vi "Write Temperature Control.lvclass.vi"(10 "Temperature Control.lvclass":refnum<class "Temperature Control.lvclass">, 11 "Measurements in":refnum<class "Measurement.lvclass">) -> (3 "Measurements out":refnum<class "Measurement.lvclass">)   [LabVIEW 2020, in "Measurement.lvclass"]
uses:
  Measurement.lvclass
  Instruments/Temperature Control/Temperature Control.lvclass
  Measurement.lvclass/Measurement.ctl
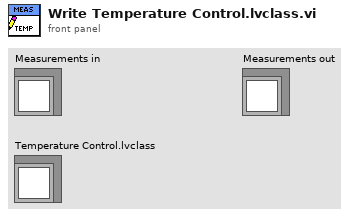
[diagram p1: front panel]
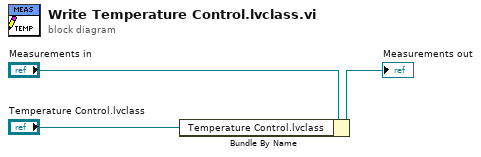
[diagram p0: block diagram]
diagram:
  n1 = Bundle By Name(cluster="Measurements in", "Temperature Control.lvclass"="Temperature Control.lvclass") -> (→"Measurements out":refnum<class "Measurement.lvclass">)
